vi "Register Block.vi"(8 "error in (no error)":errorcluster, 10 "Block Type":refnum<class "Block.lvclass">, 11 "Manager in":refnum<class "Manager.lvclass">) -> (0 "error out":errorcluster, 2 "Initialized Block":refnum<class "Block.lvclass">, 3 "Manager out":refnum<class "Manager.lvclass">)   [LabVIEW 2020, in "Parallel Block.lvlib" / "Manager.lvclass"]
uses:
  Manager.lvclass
  Manager.lvclass/Manager.ctl
  Block Command.ctl
  Block/Block.lvclass
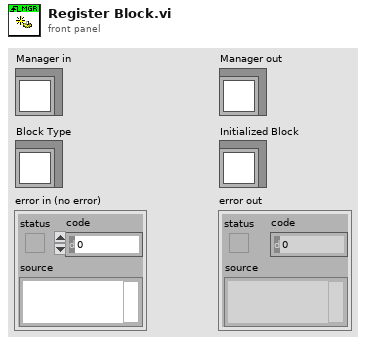
[diagram p1: front panel]
types:
  T1 = typedef "Parallel Block.lvlib/Manager.lvclass/Block Command.ctl" = enum16{"Run", "Pause", "Step", "Close"}
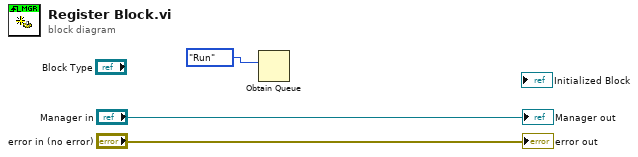
[diagram p0: block diagram]
diagram:
  n1 = Obtain Queue(element data type=Block_Command."Run" ("Block Command")) -> ()  [unwired: 4 in, 3 out]
  "error out" <- "error in (no error)"
  "Manager out" <- "Manager in"
